vi "Demo_OpenImageFile.vi"() -> ()   [LabVIEW 2024]
doc: "Read any image formats supported by QuickTime.\n\n© Ch. Salzmann, 1994-2003"
uses:
  <userlib>/ImageProcessing/QTLIB_2595_LV86/QT_Private.ctl
  <userlib>/ImageProcessing/QTLIB_2595_LV86/QT_File.ctl
panel:
  out "error out":errorcluster={"status"=FALSE, "code"=0, "source"="In ShowImageFromFile"}
  in  "Image path":path=path "quicktimelogo.gif"
  out "The image":picture caption="new picture"
  # "Read any image formats\nsupported by QuickTime\n© Ch. Salzmann, 1994-2005"
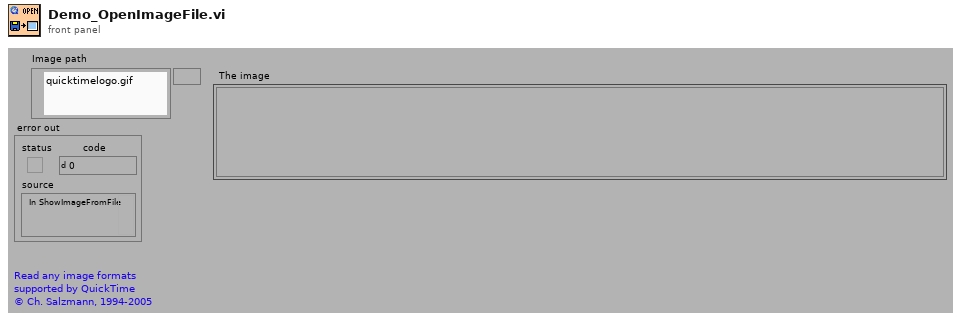
[diagram p1: front panel]
types:
  T1 = typedef "QT_File.ctl" = cluster{"Paths":string[], "Options":i32, "Dialogs":u32, "Reserved":i32}
  T2 = typedef "QT_Private.ctl" = cluster{"reserved 1":i32, "reserved 2":i32, "reserved 3":i32, "reserved 4":i32}
  T3 = typedef "QT_Image.ctl" = cluster{"Width":i32, "Height":i32, "Depth":i32, "data":u8[], "Compressed data":u8[], "Color table":u32[], "Duration":i32, "Options":i32, "Timestamp":i32, "ID":i32, "Reserved":i32, "Dialogs":u32}
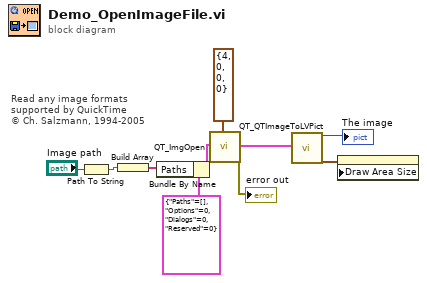
[diagram p0: block diagram]
diagram:
  # "Read any image formats\nsupported by QuickTime\n© Ch. Salzmann, 1994-2005"
  n1 = Path To String(path="Image path") -> (string=w9:string)
  n2 = Build Array(w9) -> (w1:string[])
  n3 = Bundle By Name(cluster=T1 {"Paths"=[], "Options"=0, "Dialogs"=0, "Reserved"=0} ("File Settings"), "Paths"=w1) -> (w8:T1)
  n4 = call <userlib>:"QT_ImgOpen.vi"("File Settings"=w8, "Private"=T2 {"reserved 1"=4, "reserved 2"=0, "reserved 3"=0, "reserved 4"=0}) -> ("Image Out"=w2:T3, "error out"=→"error out":errorcluster)  [unwired: 1 in, 15 out]
  n5 = call <userlib>:"QT_QTImageToLVPict.vi"("Image/Movie Out"=w2) -> ("Picture color"=→"The image":picture, "Pict Draw Area Size"=w3:cluster{"Width":i16, "Height":i16})  [unwired: 2 in, 15 out]
  n6 = property on="The image" class="Pict"("Draw Area Size"=w3) -> ()  [unwired: 2 in, 2 out]
